vi "Reinterpret U32 as I32.vi"(7 "Input":u32) -> (8 "Output":i32)   [LabVIEW 2012]
uses:
  <vilib>/rvi/FXPMathLib/FxpInterpret/XNode/nifxpmath_Interpret.xnode
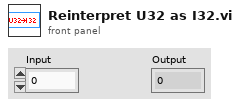
[diagram p1: front panel]
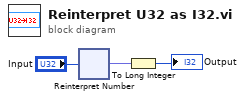
[diagram p0: block diagram]
diagram:
  n1 = xnode "Reinterpret Number"("x"="Input") -> ("y"=w3:fxp<+/-,32,32>)
  n2 = To Long Integer(number=w3) -> (32bit integer=→"Output":i32)
